vi "phase array(two antena).vi"() -> ()   [LabVIEW 2017]
panel:
  in  "오차 % (d)":dbl
  in  "Plot Color":u32(colorbox)=16715776
  in  "Grid Color":u32(colorbox)
  in  "Visible Section":u16(ring)=8
  out "2D Picture":picture
  # "Cosmetic Options"
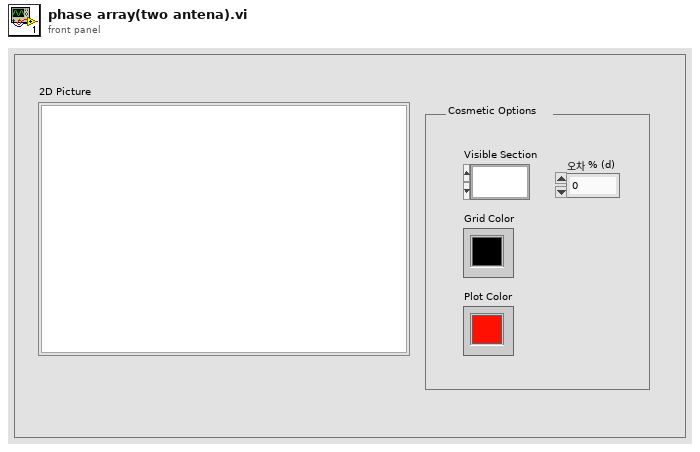
[diagram p1: front panel]
types:
  T1 = cluster{"maximum":dbl, "minimum":dbl, "clip to min":bool, "log?(F)":bool, "grid color":u32, "plot color":u32, "format and precision":cluster{"format":enum8{"Decimal", "Scientific", "Engineering", "Binary", "Octal", "Hex"}, "precision":u8}, "visible section":u16}
  T2 = typedef "LVBoundsTypeDef.ctl" = cluster{"Width":u32, "Height":u32}
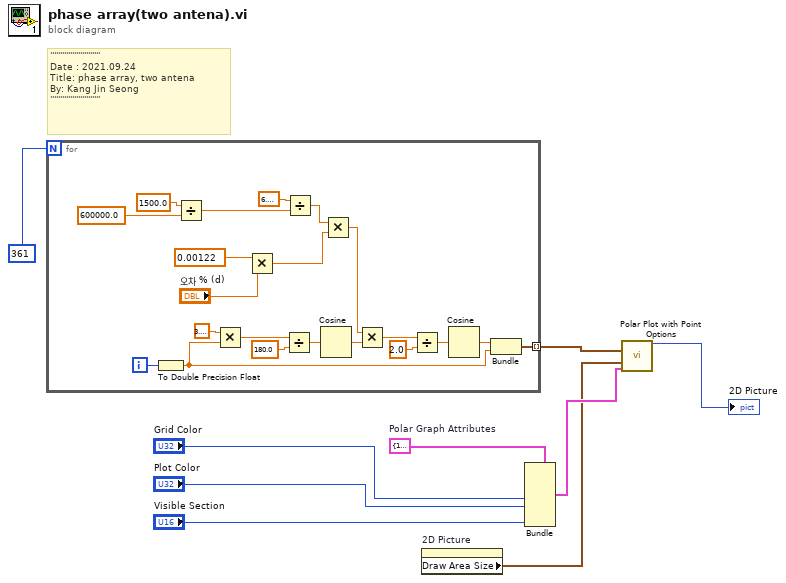
[diagram p0: block diagram]
diagram:
  w6 = T1 {"maximum"=1.0, "minimum"=0.0, "clip to min"=FALSE, "log?(F)"=FALSE, "grid color"=6710886, "plot color"=65280, "format and precision"={"format"=enum."Decimal", "precision"=1}, "visible section"=0}  # Polar Graph Attributes
  # "'''''''''''''''''''''''''\nDate : 2021.09.24\nTitle: phase array, two antena\nBy: Kang Jin Seong\n'''''''''''''''''''''''''"
  n1 = for {
    N: 361 -> [_]
    tunnel: [w20] -> w8 mode=indexing
    i -> [w29]
    n2 = To Double Precision Float(number=w29) -> (double precision float=w21:dbl)
    n3 = Divide(x=1500.0, y=600000.0) -> (x/y=w14:dbl)
    n4 = Multiply(x=3.141592653589793, y=w21) -> (x*y=w28:dbl)
    n5 = Multiply(x=0.00122 ("y"), y="오차 % (d)") -> (x*y=w10:dbl)
    n6 = Divide(x=w28, y=180.0) -> (x/y=w26:dbl)
    n7 = Divide(x=6.283185307179586, y=w14) -> (x/y=w13:dbl)
    n8 = Cosine(x=w26) -> (cos(x)=w19:dbl)
    n9 = Multiply(x=w13, y=w10) -> (x*y=w25:dbl)
    n10 = Multiply(x=w25, y=w19) -> (x*y=w24:dbl)
    n11 = Divide(x=w24, y=2.0) -> (x/y=w22:dbl)
    n12 = Cosine(x=w22) -> (cos(x)=w18:dbl)
    n13 = Bundle(w18, w21) -> (w20:cluster{dbl, dbl})  [unwired: 1 in]
  }
  n14 = property on="2D Picture" class="Pict"() -> ("Draw Area Size"=w1:T2)  [unwired: 2 in, 2 out]
  n15 = Bundle(cluster=w6, "grid color"="Grid Color", "plot color"="Plot Color", "visible section"="Visible Section") -> (w2:T1)  [unwired: 5 in]
  n16 = call <vilib>:"Polar Plot with Point Options.vi"("data array [mag, phase (deg)]"=w8, "dimensions (w,h)"=w1, "polar attributes"=w2) -> ("new picture"=→"2D Picture":picture)  [unwired: 12 in]
